vi "造波運動控制.vi"() -> ()   [LabVIEW 2014]
uses:
  <vilib>/Platform/TimedLoop/XDataNode/timing_clust.ctl
  <vilib>/Platform/TimedLoop/XDataNode/nitl_modes.ctl
  <vilib>/Platform/TimedLoop/XDataNode/wakeup.ctl
  <vilib>/Utility/file.llb/Read From Spreadsheet File (DBL).vi
  <vilib>/Utility/file.llb/Write To Spreadsheet File (DBL).vi
  <vilib>/Platform/TimedLoop/XDataNode/XDataNode.xnode
  <vilib>/Platform/TimedLoop/XDataNode/XDNodeRunTimeDep.lvlib
panel:
  out "check trajectory":cluster{"all rows":dbl[], "all rows":dbl[]}[](graph)
  out "imported data 2":cluster{"all rows":dbl[], "all rows":dbl[]}(graph)
  in  "Save file?":bool
  out "new file path (Not A Path if cancelled)":path
  in  "ORG Logic":enum32{"Low Active", "High Active"}(radio)
  in  "Home Mode":u32(ring) items=["MODE1_Abs"=0, "MODE2_Lmt "=1, "MODE3_Ref "=2, "MODE4_Abs_Ref"=3, "MODE5_Abs_NegRef "=4, "MODE6_Lmt_Ref "=5, "MODE7_AbsSearch "=6, "MODE8_LmtSearch"=7, "MODE9_AbsSearch_Ref "=8, "MODE10_AbsSearch_NegRef "=9, "MODE11_LmtSearch_Ref "=10, "MODE12_AbsSearchRefind"=11, "MODE13_LmtSearchRefind"=12, "MODE14_AbsSearchRefind_Ref"=13, "MODE15_AbsSearchRefind_NegRef"=14, "MODE16_LmtSearchRefind_Ref"=15, "CiA402_MODE1"=101, "CiA402_MODE2"=102, "CiA402_MODE3"=103, "CiA402_MODE4"=104, "CiA402_MODE5"=105, "CiA402_MODE6"=106, "CiA402_MODE7"=107, "CiA402_MODE8"=108, "CiA402_MODE9"=109, "CiA402_MODE10"=110, "CiA402_MODE11"=111, "CiA402_MODE12"=112, "CiA402_MODE13"=113, "CiA402_MODE14"=114, "CiA402_MODE15"=115, "CiA402_MODE16"=116, "CiA402_MODE17"=117, "CiA402_MODE18"=118, "CiA402_MODE19"=119, "CiA402_MODE20"=120, "CiA402_MODE21"=121, "CiA402_MODE22"=122, "CiA402_MODE23"=123, "CiA402_MODE24"=124, "CiA402_MODE25"=125, "CiA402_MODE26"=126, "CiA402_MODE27"=127, "CiA402_MODE28"=128, "CiA402_MODE29"=129, "CiA402_MODE30"=130, "CiA402_MODE31"=131, "CiA402_MODE32"=132, "CiA402_MODE33"=133, "CiA402_MODE34"=134, "CiA402_MODE35"=135, "CiA402_MODE36"=136, "CiA402_MODE37"=137]
  in  "Direction":enum32{"Negative", "Positive"}(radio)
  in  "Home":bool
  out "ORG":bool
  out "EZ":bool
  out "HLMT+":bool
  out "HLMT-":bool
  out "Waveform Chart":dbl(graph)
  out "t":dbl[](array[numeric])
  out "xi":dbl[](array[numeric]) format="%#_6f"
  out "Freespace":u16
  out "imported data":cluster{"all rows":dbl[], "all rows":dbl[]}(graph)
  in  "file path (xi)":path=path "C:/Users/NTU WAVES/Desktop/實驗操作/Nwave_Experiment_Xi.txt"
  in  "file path (t)":path=path "C:/Users/NTU WAVES/Desktop/實驗操作/Nwave_Experiment_t.txt"
  in  "import file":bool
  out "Error Code:":u32 format="%x"
  out "Error Msg":string
  out "Error":bool
  in  "Reset Error":bool
  out "Instrument":string="if you want to exit program,please press \"Exit Program\" button"
  out "DeviceNum List":u32[](array[numeric])
  out "Servo_Off":bool
  in  "Servo_On":bool
  in  "Servo On":bool
  out "Axis State:":string
  out "CloseSuccess":bool
  in  "Device Type":u16(ring) items=["PCI-1203-06AE (M0)"]
  out "Ret_GetCommandPosition":u32
  out "Exit Program":bool
  out "DeviceOpened":bool
  out "AxisOpened":bool
  out "AxisHandle_Array":u32[](array[numeric])
  out "DevAxesCount":u32
  out "EmgSucces":bool
  out "DecSuccess":bool
  in  "Stop Mode":enum32{"Dec", "Emg"}(radio)
  in  "Operate Axis":T1(radio)
  in  "Stop":bool
  in  "Move":bool
  out "ResetCounter":bool
  in  "Reset Counter":bool
  out "Axis Position":T2
  out "DeviceHandle":u32
  in  "Stop":bool
  in  "Close Board":bool
  in  "Open Board":bool
  # "Open: Open Board -Servo on\nClose:Servo  off -Close Board"
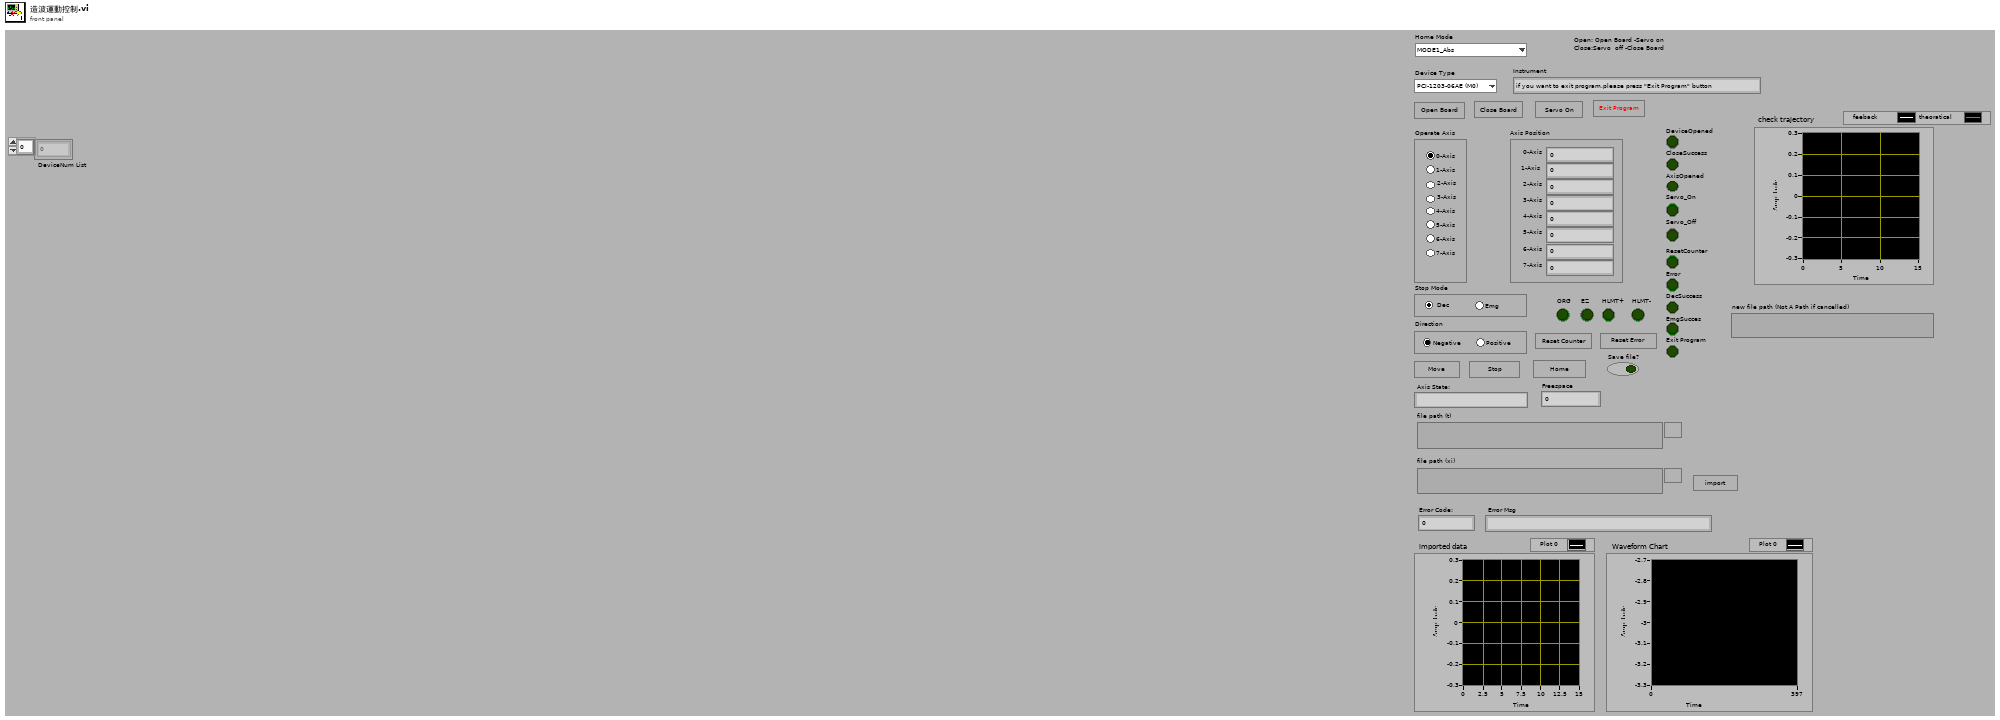
[diagram p1: front panel]
types:
  T1 = enum32{"0-Axis", "1-Axis", "2-Axis", "3-Axis", "4-Axis", "5-Axis", "6-Axis", "7-Axis"}
  T2 = cluster{"0-Axis":dbl, "1-Axis":dbl, "2-Axis":dbl, "3-Axis":dbl, "4-Axis":dbl, "5-Axis":dbl, "6-Axis":dbl, "7-Axis":dbl}
  T3 = cluster{"DeviceNum":u32, "U*8 Array":cluster{"U*8 Array[0]":u8, "U*8 Array[1]":u8, "U*8 Array[2]":u8, "U*8 Array[3]":u8, "U*8 Array[4]":u8, "U*8 Array[5]":u8, "U*8 Array[6]":u8, "U*8 Array[7]":u8, "U*8 Array[8]":u8, "U*8 Array[9]":u8, "U*8 Array[10]":u8, "U*8 Array[11]":u8, "U*8 Array[12]":u8, "U*8 Array[13]":u8, "U*8 Array[14]":u8, "U*8 Array[15]":u8, "U*8 Array[16]":u8, "U*8 Array[17]":u8, "U*8 Array[18]":u8, "U*8 Array[19]":u8, "U*8 Array[20]":u8, "U*8 Array[21]":u8, "U*8 Array[22]":u8, "U*8 Array[23]":u8, "U*8 Array[24]":u8, "U*8 Array[25]":u8, "U*8 Array[26]":u8, "U*8 Array[27]":u8, "U*8 Array[28]":u8, "U*8 Array[29]":u8, "U*8 Array[30]":u8, "U*8 Array[31]":u8, "U*8 Array[32]":u8, "U*8 Array[33]":u8, "U*8 Array[34]":u8, "U*8 Array[35]":u8, "U*8 Array[36]":u8, "U*8 Array[37]":u8, "U*8 Array[38]":u8, "U*8 Array[39]":u8, "U*8 Array[40]":u8, "U*8 Array[41]":u8, "U*8 Array[42]":u8, "U*8 Array[43]":u8, "U*8 Array[44]":u8, "U*8 Array[45]":u8, "U*8 Array[46]":u8, "U*8 Array[47]":u8, "U*8 Array[48]":u8, "U*8 Array[49]":u8}, "NumOfSubDevice":i16}[]
  T4 = cluster{"U*8 Array[0]":u8, "U*8 Array[1]":u8, "U*8 Array[2]":u8, "U*8 Array[3]":u8, "U*8 Array[4]":u8, "U*8 Array[5]":u8, "U*8 Array[6]":u8, "U*8 Array[7]":u8, "U*8 Array[8]":u8, "U*8 Array[9]":u8, "U*8 Array[10]":u8, "U*8 Array[11]":u8, "U*8 Array[12]":u8, "U*8 Array[13]":u8, "U*8 Array[14]":u8, "U*8 Array[15]":u8, "U*8 Array[16]":u8, "U*8 Array[17]":u8, "U*8 Array[18]":u8, "U*8 Array[19]":u8, "U*8 Array[20]":u8, "U*8 Array[21]":u8, "U*8 Array[22]":u8, "U*8 Array[23]":u8, "U*8 Array[24]":u8, "U*8 Array[25]":u8, "U*8 Array[26]":u8, "U*8 Array[27]":u8, "U*8 Array[28]":u8, "U*8 Array[29]":u8, "U*8 Array[30]":u8, "U*8 Array[31]":u8, "U*8 Array[32]":u8, "U*8 Array[33]":u8, "U*8 Array[34]":u8, "U*8 Array[35]":u8, "U*8 Array[36]":u8, "U*8 Array[37]":u8, "U*8 Array[38]":u8, "U*8 Array[39]":u8, "U*8 Array[40]":u8, "U*8 Array[41]":u8, "U*8 Array[42]":u8, "U*8 Array[43]":u8, "U*8 Array[44]":u8, "U*8 Array[45]":u8, "U*8 Array[46]":u8, "U*8 Array[47]":u8, "U*8 Array[48]":u8, "U*8 Array[49]":u8}
  T5 = typedef "XDNodeRunTimeDep.lvlib/timing_clust.ctl" = cluster{"Expected End [f-1]":u64, "Actual End [f-1]":u64, "Finished Late? [f-1]":bool, "Expected End [i-1]":u64, "Actual End [i-1]":u64, "Finished Late? [i-1]":bool, "Expected Start [i]":u64, "Actual Start [i]":u64, "Expected Start [f]":u64, "Actual Start [f]":u64, "Source Name":string, "Structure Name":string, "Period":i64, "Deadline":i64, "Offset":i64, "Start":i64, "Priority":i32, "Timeout":i32, "Mode":T6, "Wakeup Reason":T7, "Error":errorcluster, "Source Type":string, "Secondary Source Type":string, "Global End Time":u64, "Global Start Time":u64, "Frame Duration":u64, "Iteration Duration":u64, "Assigned CPU":i32, "I/O Scan Engine Mode":u32}
  T6 = typedef "XDNodeRunTimeDep.lvlib/nitl_modes.ctl" = enum32{"No Change", "Process missed periods, maintain original phase", "Discard missed periods, maintain original phase", "Process missed periods, ignore original phase", "Discard missed periods, ignore original phase"}
  T7 = typedef "XDNodeRunTimeDep.lvlib/wakeup.ctl" = enum32{"Normal", "Aborted", "Asynchronous wakeup", "Timing source error", "Timed loop error", "Timeout"}
  T8 = cluster{"[0]":dbl, "[1]":dbl, "[2]":dbl, "[3]":dbl, "[4]":dbl, "[5]":dbl, "[6]":dbl, "[7]":dbl}
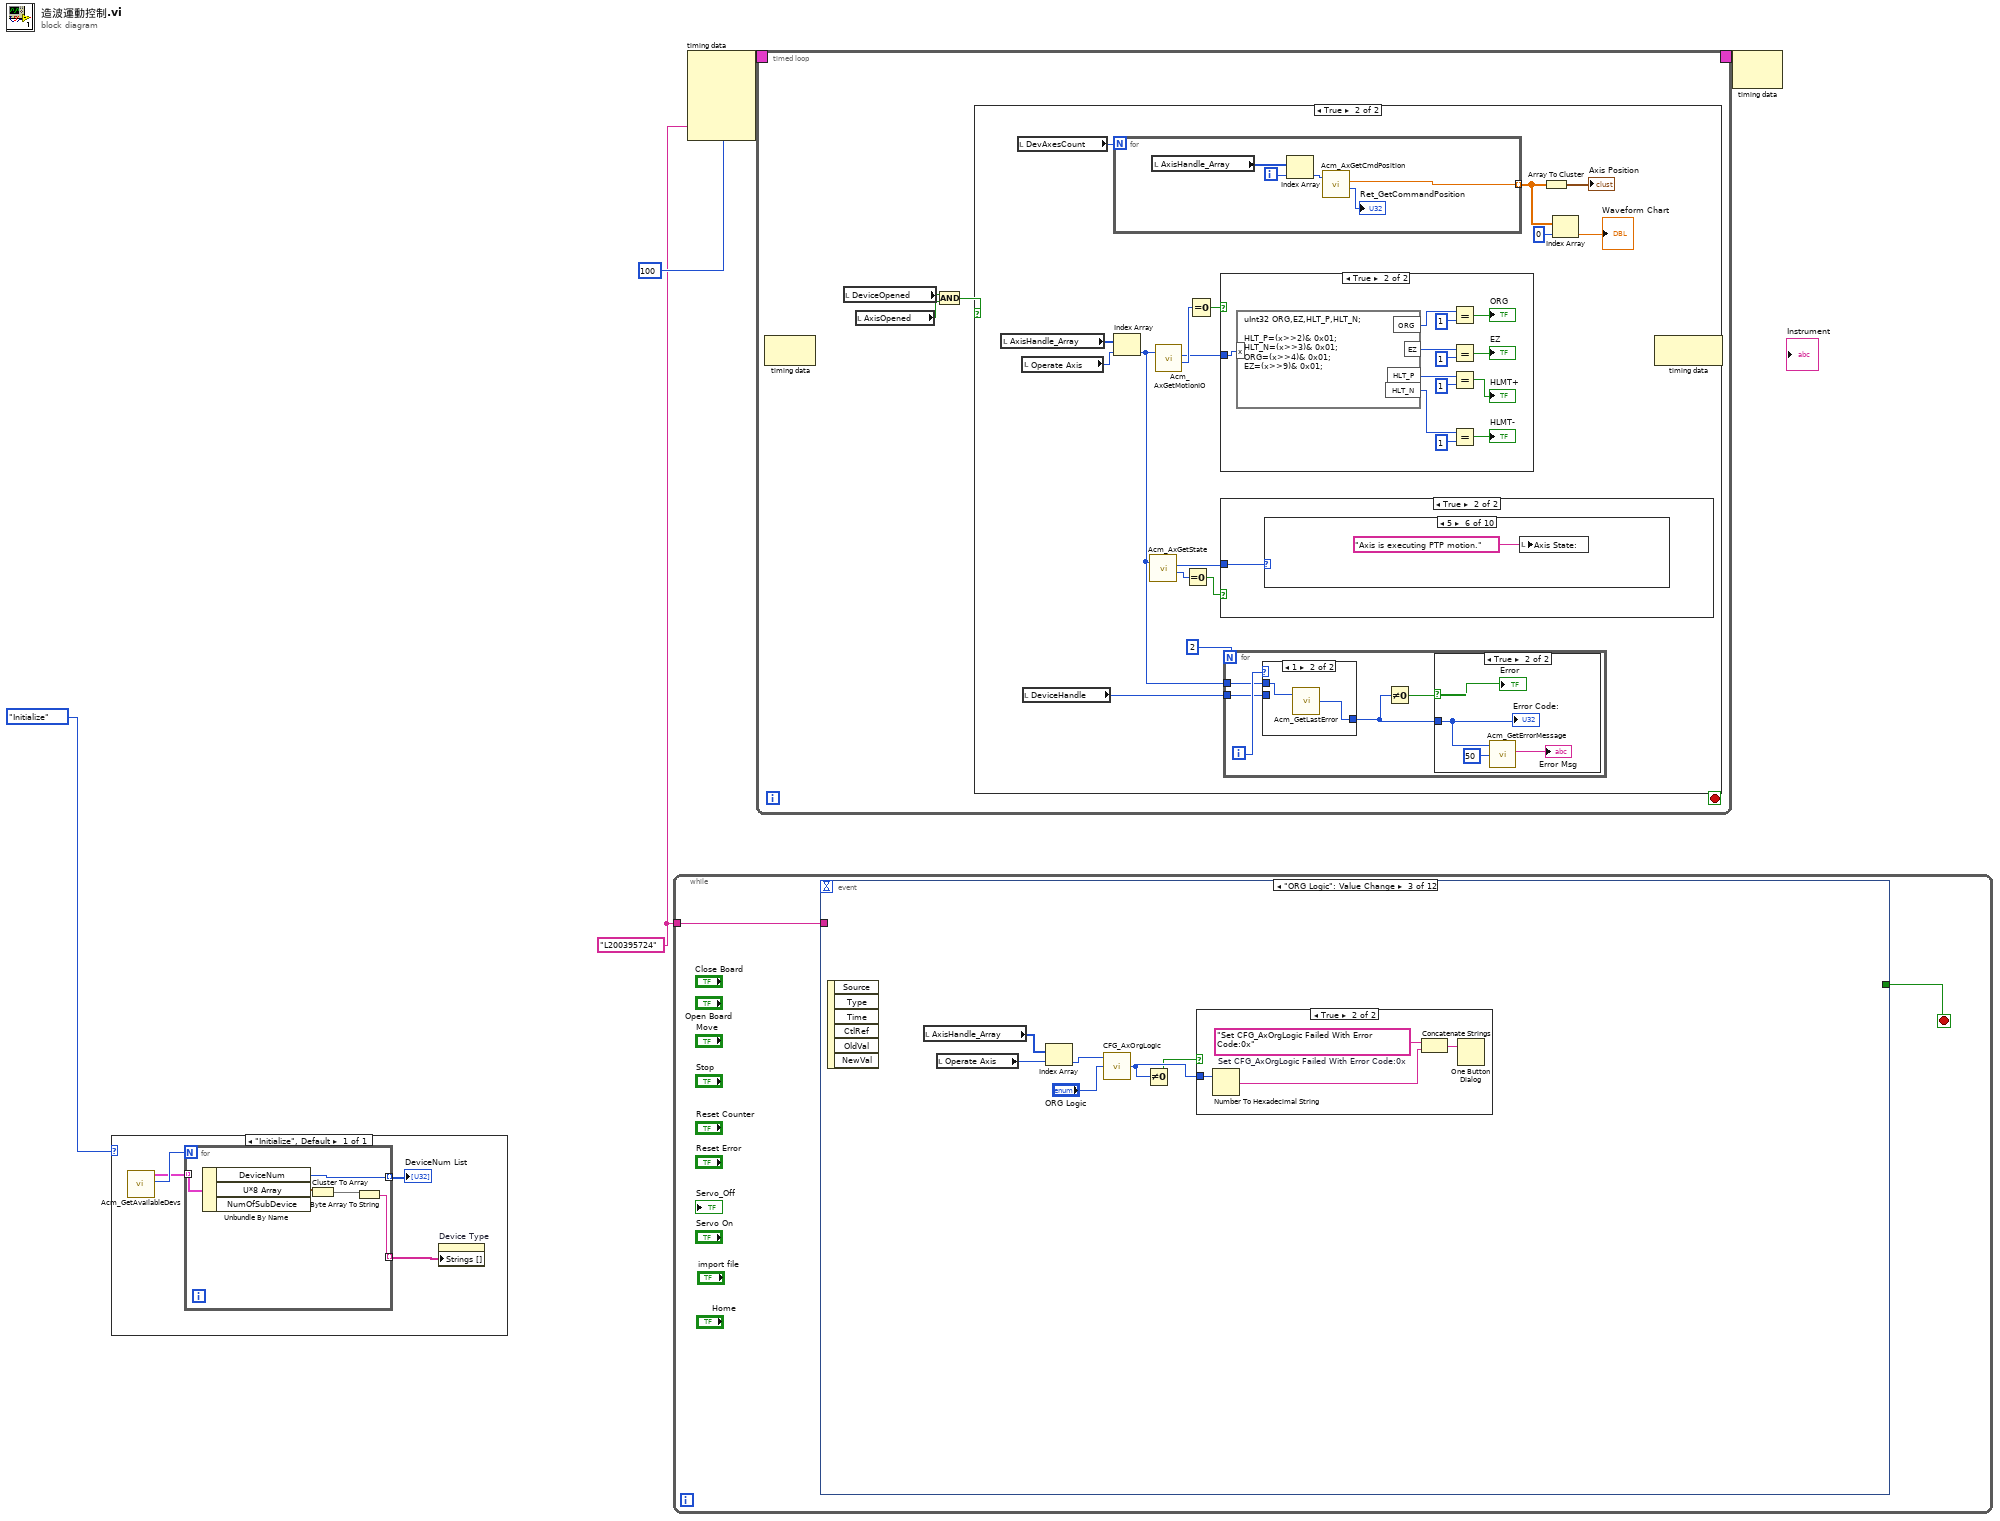
[diagram p0: block diagram]
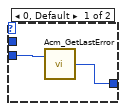
[diagram p5: hidden frame]
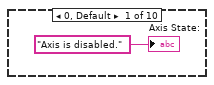
[diagram p7: hidden frame]
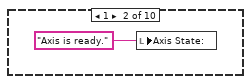
[diagram p8: hidden frame]
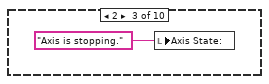
[diagram p9: hidden frame]
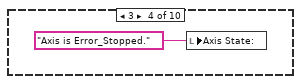
[diagram p10: hidden frame]
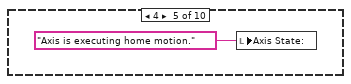
[diagram p11: hidden frame]
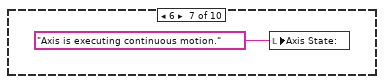
[diagram p12: hidden frame]
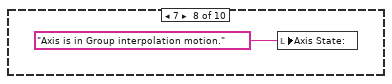
[diagram p13: hidden frame]
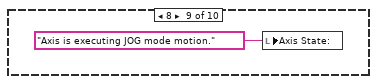
[diagram p14: hidden frame]
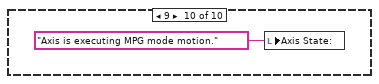
[diagram p15: hidden frame]
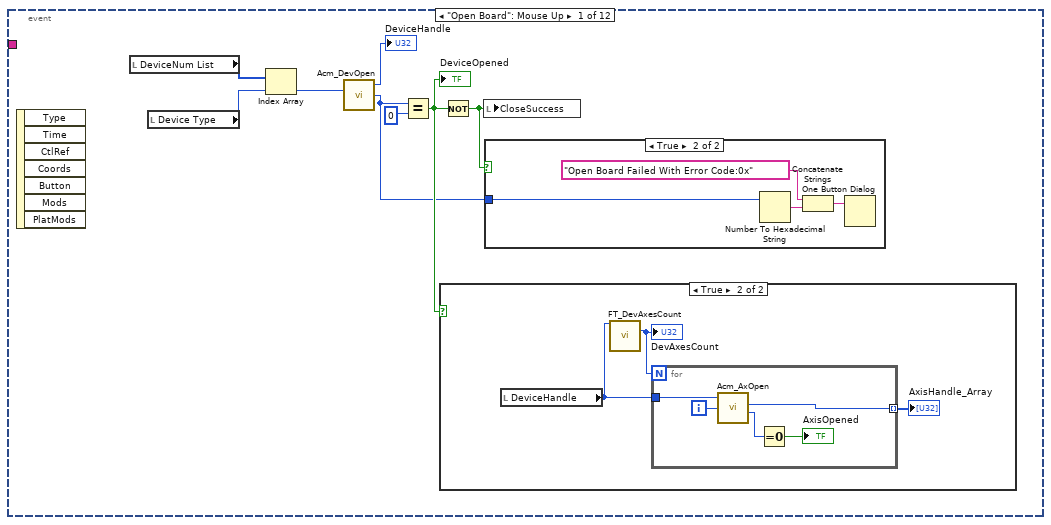
[diagram p16: hidden frame]
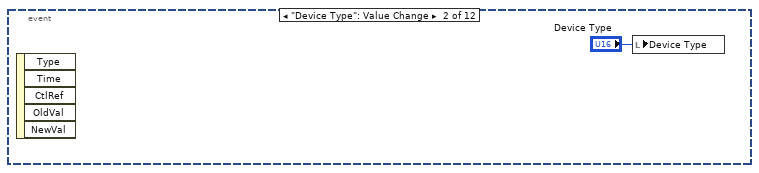
[diagram p19: hidden frame]
diagram:
  w2 = "L200395724" ("结构名称")
  n1 = case shown="\"Initialize\", Default" enum16{"Initialize"}."Initialize" ("Enum") {
    frame "Initialize", Default {
      n2 = call <userlib>:"Acm_GetAvailableDevs.vi"() -> ("DeviceList"=w8:T3, "OutEntries"=w9:u32)  [unwired: 1 in, 4 out]
      n3 = for {
        N: w9 -> [_]
        tunnel: w8 -> [w14] mode=indexing
        tunnel: [w11] -> w7 mode=indexing
        tunnel: [w10] -> w6 mode=indexing
        n4 = Unbundle By Name(w14) -> ("DeviceNum"=w11:u32, "U*8 Array"=w13:T4)  [unwired: 1 out]
        n5 = Cluster To Array(cluster=w13) -> (array=w12:u8[])
        n6 = Byte Array To String(unsigned byte array=w12) -> (string=w10:string)
      }
      "DeviceNum List" <- w7
      n7 = property on="Device Type" class="Ring (strict)"("Strings []"=w6) -> ()  [unwired: 2 in, 2 out]
    }
  }
  n8 = while {
    tunnel: w2 -> [w15]
    stop <- w16 stop-if-true
    n9 = event shown="[2] \"ORG Logic\": Value Change" {
      selector: _ -> [_ _ _ _ _ _ _ _ _ _ _ _]
      dyn-events: _ -> [_ _ _ _ _ _ _ _ _ _ _ _]
      timeout: _ -> [_ _ _ _ _ _ _ _ _ _ _ _]
      tunnel: [_ _ _ _ _ _ _ _ _ _ _ "Stop"] -> w16
      tunnel: w15 -> [_ _ _ _ _ _ _ _ _ _ _ w216]
      event "Open Board": Mouse Up {
        n10 = event-data() -> ()  [unwired: 8 out]
        n11 = local read "DeviceNum List"() -> (w19:u32[])
        n12 = local read "Device Type"() -> (w18:u16)
        n13 = Index Array(array=w19, index=w18) -> (element=w17:u32)
        n14 = call <userlib>:"Acm_DevOpen.vi"("DeviceNumber"=w17) -> ("ReturnValue"=w21:u32, "DeviceHandle"=→"DeviceHandle":u32)  [unwired: 1 in, 1 out]
        n15 = Equal?(x=w21, y=u32 0) -> (x = y?=w22:bool)
        "DeviceOpened" <- w22
        n16 = case shown="True" w22 {
          frame False {
          }
          frame True {
            n17 = local read "DeviceHandle"() -> (w30:u32)
            n18 = call <userlib>:"FT_DevAxesCount.vi"("Handle"=w30) -> ("DevAxesCount"=w31:u32)  [unwired: 1 in, 13 out]
            "DevAxesCount" <- w31
            n19 = for {
              N: w31 -> [_]
              tunnel: w30 -> [w36]
              tunnel: [w32] -> w29 mode=indexing
              i -> [w35]
              n20 = call <userlib>:"Acm_AxOpen.vi"("PhyAxis"=w35, "DeviceHandle"=w36) -> ("ReturnValue"=w34:u32, "AxisHandle"=w32:u32)  [unwired: 1 in, 2 out]
              n21 = Equal To 0?(x=w34) -> (x = 0?=→"AxisOpened":bool)
            }
            "AxisHandle_Array" <- w29
          }
        }
        n22 = Not(x=w22) -> (.not. x?=w20:bool)
        n23 = local write "CloseSuccess"(w20) -> ()
        n24 = case shown="True" w20 {
          tunnel: w21 -> [_ w28]
          frame False {
          }
          frame True {
            n25 = Number To Hexadecimal String(2:w28) -> (0:w26:string)  [unwired: 1 out]
            n26 = Concatenate Strings("Open Board Failed With Error Code:0x", w26) -> (w25:string)
            n27 = One Button Dialog(message=w25) -> ()  [unwired: 2 out]
          }
        }
      }
      event "Device Type": Value Change {
        n28 = event-data() -> ()  [unwired: 6 out]
        n29 = local write "Device Type"("Device Type") -> ()
      }
      event "ORG Logic": Value Change {
        n30 = event-data() -> ()  [unwired: 7 out]
        n31 = local read "AxisHandle_Array"() -> (w42:u32[])
        n32 = local read "Operate Axis"() -> (w41:T1)
        n33 = Index Array(array=w42, index=w41) -> (element=w40:u32)
        n34 = call <userlib>:"CFG_AxOrgLogic.vi"("CFG_AxOrgLogic"="ORG Logic", "Handle"=w40) -> ("ReturnValue"=w39:u32)  [unwired: 1 in, 2 out]
        n35 = Not Equal To 0?(x=w39) -> (x != 0?=w38:bool)
        n36 = case shown="True" w38 {
          tunnel: w39 -> [_ w44]
          frame False {
          }
          frame True {
            w47 = "Set CFG_AxOrgLogic Failed With Error Code:0x"  # Set CFG_AxOrgLogic Failed With Error Code:0x
            n37 = Number To Hexadecimal String(2:w44) -> (0:w46:string)  [unwired: 1 out]
            n38 = Concatenate Strings(w47, w46) -> (w45:string)
            n39 = One Button Dialog(message=w45) -> ()  [unwired: 2 out]
          }
        }
      }
      event "Servo On": Value Change {
        n40 = event-data() -> ()  [unwired: 6 out]
        n41 = local read "AxisHandle_Array"() -> (w57:u32[])
        n42 = local read "Operate Axis"() -> (w56:T1)
        n43 = case shown="True" "Servo_On" {
          tunnel: [u32 1 u32 0] -> w54
          frame False {
          }
          frame True {
          }
        }
        n44 = Index Array(array=w57, index=w56) -> (element=w55:u32)
        n45 = call <userlib>:"Acm_AxSetSvOn.vi"("OnOff"=w54, "AxisHandle"=w55) -> ("ReturnValue"=w48:u32)  [unwired: 1 in, 2 out]
        n46 = local read "Servo On"() -> (w51:bool)
        n47 = Not Equal To 0?(x=w48) -> (x != 0?=w53:bool)
        n48 = Not(x=w53) -> (.not. x?=w52:bool)
        n49 = case shown="True" w53 {
          tunnel: w48 -> [_ w62]
          frame False {
          }
          frame True {
            w65 = "Servo On/Off Failed With Error Code:0x"  # Servo On/Off Failed With Error Code:0x
            n50 = Number To Hexadecimal String(2:w62) -> (0:w64:string)  [unwired: 1 out]
            n51 = Concatenate Strings(w65, w64) -> (w63:string)
            n52 = One Button Dialog(message=w63) -> ()  [unwired: 2 out]
          }
        }
        n53 = And(x=w51, y=w52) -> (x .and. y?=w50:bool)
        n54 = case shown="True" w50 {
          frame False {
            n55 = local write "Servo_On"(FALSE ("Servo_On")) -> ()
            n56 = local write "Servo_Off"(TRUE ("Servo_Off")) -> ()
          }
          frame True {
            n57 = local write "Servo_On"(TRUE ("Servo_On")) -> ()
            n58 = local write "Servo_Off"(FALSE ("Servo_Off")) -> ()
          }
        }
      }
      event "import file": Mouse Up {
        n59 = event-data() -> ()  [unwired: 9 out]
        n60 = local read "AxisHandle_Array"() -> (w85:u32[])
        n61 = local read "Operate Axis"() -> (w69:T1)
        n62 = call-poly <vilib>:"Read From Spreadsheet File.vi"("number of rows (all:-1)"=-1, "file path (dialog if empty)"="file path (t)") -> ("all rows"=w80:dbl[][])  [unwired: 5 in, 4 out]
        n63 = call-poly <vilib>:"Read From Spreadsheet File.vi"("number of rows (all:-1)"=-1, "file path (dialog if empty)"="file path (xi)") -> ("all rows"=w78:dbl[][])  [unwired: 5 in, 4 out]
        n64 = Index Array(array=w85, index=w69) -> (element=w76:u32)
        n65 = Index Array(array=w80, index (col)=0 ("disabled index (col)")) -> (element=w71:dbl[])  [unwired: 1 in]
        "t" <- w71
        n66 = Index Array(array=w78, index (col)=0 ("disabled index (col)")) -> (element=w70:dbl[])  [unwired: 1 in]
        "xi" <- w70
        n67 = call <userlib>:"Acm_AxCheckPTBuffer.vi"("AxisHandle"=w76) -> ("Freespace"=→"Freespace":u16, "ReturnValue"=w74:u32)  [unwired: 1 in, 2 out]
        n68 = Equal To 0?(x=w74) -> (x = 0?=w73:bool)
        n69 = Bundle("all rows"=w71, "all rows"=w70) -> (→"imported data":cluster{"all rows":dbl[], "all rows":dbl[]})  [unwired: 1 in]
        n70 = Not(x=w73) -> (.not. x?=w72:bool)
        n71 = case shown="True" w72 {
          tunnel: w74 -> [_ w86]
          frame False {
          }
          frame True {
            n72 = Number To Hexadecimal String(2:w86) -> (0:w88:string)  [unwired: 1 out]
            n73 = Concatenate Strings("PTBuffer Absolutely Failed With Error Code:0x", w88) -> (w87:string)
            n74 = One Button Dialog(message=w87) -> ()  [unwired: 2 out]
          }
        }
      }
      event "Move": Mouse Up {
        n75 = event-data() -> ()  [unwired: 9 out]
        n76 = local read "AxisHandle_Array"() -> (w112:u32[])
        n77 = local read "t"() -> (w100:dbl[])
        n78 = local read "xi"() -> (w111:dbl[])
        n79 = Index Array(array=w112, index="Operate Axis") -> (element=w104:u32)
        n80 = Multiply(x=w100, y=1000) -> (x*y=w95:dbl[])
        n81 = Multiply(x=100000, y=w111) -> (x*y=w96:dbl[])
        n82 = Bundle(w95, w96) -> (→"imported data 2":cluster{dbl[], dbl[]})  [unwired: 1 in]
        n83 = Tick Count (ms)() -> (millisecond timer value=w105:u32)
        n84 = for {
          tunnel: w104 -> [w137]
          tunnel: w96 -> [w136] mode=indexing
          tunnel: w95 -> [w135] mode=indexing
          n85 = call <userlib>:"Acm_AxAddPTData.vi"("Time"=w135, "Position"=w136, "AxisHandle"=w137) -> ("AxisHandle"=w138:u32)  [unwired: 1 in, 2 out]
          n86 = call <userlib>:"Acm_AxStartPT.vi"("AxisHandle"=w138) -> ()  [unwired: 2 in, 3 out]
        }
        n87 = Array Size(array=w100) -> (size(s)=w107:i32)
        n88 = Decrement(x=w107) -> (x-1=w106:i32)
        n89 = Index Array(array=w95, index=w106) -> (element=w102:dbl)
        n90 = while {
          tunnel: w102 -> [w131]
          shift-right: [w129] -> w93
          shift-left: dbl[] [] -> [w130]
          tunnel: w105 -> [w127]
          tunnel: w104 -> [w126]
          shift-right: [w125] -> w94
          shift-left: dbl[] [] -> [w124]
          i -> [w123]
          stop <- w133 stop-if-true
          w122 = u32 10 ("millisecond multiple")
          n91 = call <userlib>:"Acm_AxGetActualPosition.vi"("AxisHandle"=w126) -> ("Position"=w128:dbl)  [unwired: 1 in, 3 out]
          n92 = Multiply(x=w123, y=w122) -> (x*y=w120:u32)
          n93 = Tick Count (ms)() -> (millisecond timer value=w134:u32)
          n94 = Divide(x=w128, y=100000.0) -> (x/y=w118:dbl)
          n95 = Divide(x=w120, y=u32 1000) -> (x/y=w121:dbl)
          n96 = Subtract(x=w134, y=w127) -> (x-y=w132:u32)
          n97 = Wait Until Next ms Multiple(millisecond multiple=w122) -> ()  [unwired: 1 out]
          n98 = Insert Into Array(array=w130, new element=w118) -> (w129:dbl[])  [unwired: 1 in]
          n99 = Greater Or Equal?(x=w132, y=w131) -> (x >= y?=w133:bool)
          n100 = Insert Into Array(array=w124, new element=w121) -> (w125:dbl[])  [unwired: 1 in]
        }
        n101 = local read "imported data"() -> (w91:cluster{"all rows":dbl[], "all rows":dbl[]})
        n102 = Build Array(w94, w93) -> (w98:dbl[][])
        n103 = Bundle(w94, w93) -> (w92:cluster{dbl[], dbl[]})  [unwired: 1 in]
        n104 = case shown="True" "Save file?" {
          tunnel: w98 -> [_ w115]
          frame False {
          }
          frame True {
            n105 = call-poly <vilib>:"Write To Spreadsheet File.vi"("delimiter (\\t)"="," ("delimiter (\\t)"), "transpose? (no:F)"=TRUE, "2D data"=w115) -> ("new file path (Not A Path if cancelled)"=→"new file path (Not A Path if cancelled)":path)  [unwired: 5 in]
          }
        }
        n106 = Build Array(w92, w91) -> (→"check trajectory":cluster{"all rows":dbl[], "all rows":dbl[]}[])
      }
      event "Stop": Mouse Up {
        n107 = event-data() -> ()  [unwired: 8 out]
        n108 = local read "AxisHandle_Array"() -> (w142:u32[])
        n109 = local read "Operate Axis"() -> (w140:T1)
        n110 = Index Array(array=w142, index=w140) -> (element=w141:u32)
        n111 = case shown="\"Emg\"" "Stop Mode" {
          tunnel: w141 -> [w145 w154]
          frame "Dec", Default {
            n112 = call <userlib>:"Acm_AxStopDec.vi"("AxisHandle"=w145) -> ("ReturnValue"=w146:u32)  [unwired: 1 in, 2 out]
            n113 = Equal To 0?(x=w146) -> (x = 0?=w144:bool)
            "DecSuccess" <- w144
            n114 = Not(x=w144) -> (.not. x?=w143:bool)
            n115 = case shown="True" w143 {
              tunnel: w145 -> [_ w150]
              frame False {
              }
              frame True {
                n116 = Number To Hexadecimal String(2:w150) -> (0:w148:string)  [unwired: 1 out]
                n117 = Concatenate Strings("Stop Failed With Error Code:0x", w148) -> (w147:string)
                n118 = One Button Dialog(message=w147) -> ()  [unwired: 2 out]
              }
            }
          }
          frame "Emg" {
            n119 = call <userlib>:"Acm_AxStopEmg.vi"("AxisHandle"=w154) -> ("ReturnValue"=w151:u32)  [unwired: 1 in, 2 out]
            n120 = Equal To 0?(x=w151) -> (x = 0?=w153:bool)
            "EmgSucces" <- w153
            n121 = Not(x=w153) -> (.not. x?=w152:bool)
            n122 = case shown="True" w152 {
              tunnel: w151 -> [_ w158]
              frame False {
              }
              frame True {
                n123 = Number To Hexadecimal String(2:w158) -> (0:w156:string)  [unwired: 1 out]
                n124 = Concatenate Strings("Stop failed with Error Code:0x", w156) -> (w155:string)
                n125 = One Button Dialog(message=w155) -> ()  [unwired: 2 out]
              }
            }
          }
        }
      }
      event "Home": Mouse Up {
        n126 = event-data() -> ()  [unwired: 9 out]
        n127 = local read "AxisHandle_Array"() -> (w161:u32[])
        n128 = local read "Operate Axis"() -> (w160:T1)
        n129 = Index Array(array=w161, index=w160) -> (element=w159:u32)
        n130 = case shown="\"Positive\"" "Direction" {
          tunnel: w159 -> [w163 w173]
          frame "Negative", Default {
            n131 = call <userlib>:"Acm_AxHome.vi"("DirMode"=u32 1, "HomeMode"="Home Mode", "AxisHandle"=w163) -> ("ReturnValue"=w166:u32)  [unwired: 1 in, 2 out]
            n132 = Equal To 0?(x=w166) -> (x = 0?=w167:bool)
            n133 = Not(x=w167) -> (.not. x?=w168:bool)
            n134 = case shown="True" w168 {
              tunnel: w166 -> [_ w169]
              frame False {
              }
              frame True {
                n135 = Number To Hexadecimal String(2:w169) -> (0:w171:string)  [unwired: 1 out]
                n136 = Concatenate Strings("Go Home failed with Error Code:0x", w171) -> (w170:string)
                n137 = One Button Dialog(message=w170) -> ()  [unwired: 2 out]
              }
            }
          }
          frame "Positive" {
            n138 = local read "Home Mode"() -> (w175:u32)
            n139 = call <userlib>:"Acm_AxHome.vi"("DirMode"=u32 0, "HomeMode"=w175, "AxisHandle"=w173) -> ("ReturnValue"=w177:u32)  [unwired: 1 in, 2 out]
            n140 = Not Equal To 0?(x=w177) -> (x != 0?=w176:bool)
            n141 = case shown="True" w176 {
              tunnel: w177 -> [_ w178]
              frame False {
              }
              frame True {
                n142 = Number To Hexadecimal String(2:w178) -> (0:w180:string)  [unwired: 1 out]
                n143 = Concatenate Strings("Go Home Failed With Error Code:0x", w180) -> (w179:string)
                n144 = One Button Dialog(message=w179) -> ()  [unwired: 2 out]
              }
            }
          }
        }
      }
      event "Reset Counter": Mouse Up {
        n145 = event-data() -> ()  [unwired: 8 out]
        n146 = local read "AxisOpened"() -> (w182:bool)
        n147 = case shown="True" w182 {
          frame False {
          }
          frame True {
            n148 = local read "DevAxesCount"() -> (w183:u32)
            n149 = for {
              N: w183 -> [_]
              i -> [w188]
              n150 = local read "AxisHandle_Array"() -> (w189:u32[])
              n151 = Index Array(array=w189, index=w188) -> (element=w187:u32)
              n152 = call <userlib>:"Acm_AxSetCmdPosition.vi"("Position"=0.0, "AxisHandle"=w187) -> ("ReturnValue"=w185:u32)  [unwired: 1 in, 2 out]
              n153 = Equal To 0?(x=w185) -> (x = 0?=→"ResetCounter":bool)
            }
          }
        }
      }
      event "Reset Error": Mouse Up {
        n154 = event-data() -> ()  [unwired: 9 out]
        n155 = local read "AxisOpened"() -> (w190:bool)
        n156 = case shown="True" w190 {
          frame False {
          }
          frame True {
            n157 = local read "AxisHandle_Array"() -> (w193:u32[])
            n158 = local read "Operate Axis"() -> (w191:T1)
            n159 = Index Array(array=w193, index=w191) -> (element=w192:u32)
            n160 = call <userlib>:"Acm_AxResetError.vi"("AxisHandle"=w192) -> ()  [unwired: 1 in, 3 out]
          }
        }
      }
      event "Close Board": Mouse Up {
        n161 = event-data() -> ()  [unwired: 8 out]
        n162 = stacked-sequence {
          frame #0 {
            n163 = local read "DevAxesCount"() -> (w194:u32)
            n164 = for {
              N: w194 -> [_]
              i -> [w199]
              n165 = local read "AxisHandle_Array"() -> (w200:u32[])
              n166 = Index Array(array=w200, index=w199) -> (element=w198:u32)
              n167 = call <userlib>:"Acm_AxClose.vi"("AxisHandle"=w198) -> ("ReturnValue"=w197:u32)  [unwired: 1 in, 1 out]
              n168 = Equal To 0?(x=w197) -> (x = 0?=w196:bool)
              n169 = Not(x=w196) -> (.not. x?=w195:bool)
              n170 = local write "AxisOpened"(w195) -> ()
            }
          }
          frame #1 {
            n171 = local read "DeviceHandle"() -> (w204:u32)
            n172 = call <userlib>:"Acm_DevClose.vi"("DeviceHandle"=w204) -> ("ReturnValue"=w203:u32)  [unwired: 1 in, 3 out]
            n173 = Equal To 0?(x=w203) -> (x = 0?=w202:bool)
            "CloseSuccess" <- w202
            n174 = Not(x=w202) -> (.not. x?=w201:bool)
            n175 = case shown="True" w202 {
              tunnel: w202 -> [_ w210]
              frame False {
              }
              frame True {
                n176 = Not(x=w210) -> (.not. x?=w209:bool)
                n177 = local write "DevAxesCount"(u32 0 ("DevAxesCount")) -> ()
                n178 = local write "DeviceHandle"(u32 0 ("DeviceHandle")) -> ()
                n179 = local write "DeviceOpened"(w209) -> ()
                n180 = local write "EmgSucces"(w209) -> ()
                n181 = local write "DecSuccess"(w209) -> ()
                n182 = local write "ResetCounter"(w209) -> ()
                n183 = local read "DevAxesCount"() -> (w213:u32)
                n184 = Initialize Array(u32 0 ("元素"), w213) -> (w212:u32[])
                n185 = local write "AxisHandle_Array"(w212) -> ()
              }
            }
            n186 = case shown="True" w201 {
              tunnel: w203 -> [_ w208]
              frame False {
              }
              frame True {
                n187 = Number To Hexadecimal String(2:w208) -> (0:w206:string)  [unwired: 1 out]
                n188 = Concatenate Strings("Close Board Failed With Error Code:0x", w206) -> (w205:string)
                n189 = One Button Dialog(message=w205) -> ()  [unwired: 2 out]
              }
            }
          }
        }
      }
      event "Stop": Value Change {
        n190 = event-data() -> ()  [unwired: 6 out]
        n191 = call <vilib>:"Stop Timed Structure.vi"("name"=w216) -> ()  [unwired: 2 in, 9 out]
        "Exit Program" <- "Stop"
      }
    }
  }
  n192 = node-c288(i64 100 ("周期"), w2) -> (w5:T5)  [unwired: 3 out]
  n193 = timed-loop {
    timing: w5 -> [_]
    timing-out: [_] -> w4
    stop <- _ stop-if-true
    n194 = node-c288() -> ()  [unwired: 2 out]
    n195 = local read "DeviceOpened"() -> (w219:bool)
    n196 = local read "AxisOpened"() -> (w220:bool)
    n197 = And(x=w219, y=w220) -> (x .and. y?=w218:bool)
    n198 = case shown="True" w218 {
      frame False {
      }
      frame True {
        n199 = local read "AxisHandle_Array"() -> (w234:u32[])
        n200 = local read "DevAxesCount"() -> (w235:u32)
        n201 = local read "Operate Axis"() -> (w233:T1)
        n202 = local read "DeviceHandle"() -> (w228:u32)
        n203 = for {
          N: w235 -> [_]
          tunnel: [w275] -> w227 mode=indexing
          i -> [w277]
          n204 = local read "AxisHandle_Array"() -> (w278:u32[])
          n205 = Index Array(array=w278, index=w277) -> (element=w276:u32)
          n206 = call <userlib>:"Acm_AxGetCmdPosition.vi"("AxisHandle"=w276) -> ("ReturnValue"=→"Ret_GetCommandPosition":u32, "Position"=w275:dbl)  [unwired: 1 in, 2 out]
        }
        n207 = Index Array(array=w234, index=w233) -> (element=w224:u32)
        n208 = call <userlib>:"Acm_AxGetState.vi"("AxisHandle"=w224) -> ("ReturnValue"=w232:u32, "Status"=w230:u16)  [unwired: 1 in, 2 out]
        n209 = call <userlib>:"Acm_AxGetMotionIO.vi"("AxisHandle"=w224) -> ("ReturnValue"=w222:u32, "Status"=w221:u32)  [unwired: 1 in, 2 out]
        n210 = Equal To 0?(x=w232) -> (x = 0?=w231:bool)
        n211 = Equal To 0?(x=w222) -> (x = 0?=w223:bool)
        n212 = case shown="True" w223 {
          tunnel: w221 -> [_ w237]
          frame False {
          }
          frame True {
            n213 = formula code="uInt32 ORG,EZ,HLT_P,HLT_N;\n\nHLT_P=(x>>2)& 0x01;\nHLT_N=(x>>3)& 0x01;\nORG=(x>>4)& 0x01;\nEZ=(x>>9)& 0x01;"("x"=w237) -> ("ORG"=w248:u32, "EZ"=w246:u32, "HLT_P"=w244:u32, "HLT_N"=w239:u32)
            n214 = Equal?(x=w248, y=u32 1) -> (x = y?=→"ORG":bool)
            n215 = Equal?(x=w246, y=u32 1) -> (x = y?=→"EZ":bool)
            n216 = Equal?(x=w244, y=u32 1) -> (x = y?=→"HLMT+":bool)
            n217 = Equal?(x=w239, y=u32 1) -> (x = y?=→"HLMT-":bool)
          }
        }
        n218 = case shown="True" w231 {
          tunnel: w230 -> [_ w263]
          frame False {
          }
          frame True {
            n219 = case shown="5" w263 {
              frame 0, Default {
                "Axis State:" <- "Axis is disabled." ("Axis State:")
              }
              frame 1 {
                n220 = local write "Axis State:"("Axis is ready." ("Axis State:")) -> ()
              }
              frame 2 {
                n221 = local write "Axis State:"("Axis is stopping." ("Axis State:")) -> ()
              }
              frame 3 {
                n222 = local write "Axis State:"("Axis is Error_Stopped." ("Axis State:")) -> ()
              }
              frame 4 {
                n223 = local write "Axis State:"("Axis is executing home motion." ("Axis State:")) -> ()
              }
              frame 5 {
                n224 = local write "Axis State:"("Axis is executing PTP motion." ("Axis State:")) -> ()
              }
              frame 6 {
                n225 = local write "Axis State:"("Axis is executing continuous motion." ("Axis State:")) -> ()
              }
              frame 7 {
                n226 = local write "Axis State:"("Axis is in Group interpolation motion." ("Axis State:")) -> ()
              }
              frame 8 {
                n227 = local write "Axis State:"("Axis is executing JOG mode motion." ("Axis State:")) -> ()
              }
              frame 9 {
                n228 = local write "Axis State:"("Axis is executing MPG mode motion." ("Axis State:")) -> ()
              }
            }
          }
        }
        n229 = for {
          N: 2 -> [_]
          tunnel: w228 -> [w253]
          tunnel: w224 -> [w252]
          i -> [w254]
          n230 = case shown="1" w254 {
            tunnel: [w260 w262] -> w251
            tunnel: w253 -> [w259 _]
            tunnel: w252 -> [_ w261]
            frame 0, Default {
              n231 = call <userlib>:"Acm_GetLastError.vi"("ObjectHandle"=w259) -> ("ReturnValue"=w260:u32)  [unwired: 1 in, 2 out]
            }
            frame 1 {
              n232 = call <userlib>:"Acm_GetLastError.vi"("ObjectHandle"=w261) -> ("ReturnValue"=w262:u32)  [unwired: 1 in, 2 out]
            }
          }
          n233 = Not Equal To 0?(x=w251) -> (x != 0?=w250:bool)
          n234 = case shown="True" w250 {
            selector: w250 -> [_ w257]
            tunnel: w251 -> [_ w256]
            frame False {
            }
            frame True {
              n235 = call <userlib>:"Acm_GetErrorMessage.vi"("nMaxError"=50, "ErrorCode"=w256) -> ("ErrorMsg"=→"Error Msg":string)  [unwired: 4 out]
              "Error" <- w257
              "Error Code:" <- w256
            }
          }
        }
        n236 = Array To Cluster(array=w227) -> (cluster=→"Axis Position":T8)
        n237 = Index Array(array=w227, index=0) -> (element=→"Waveform Chart":dbl)
      }
    }
    n238 = node-c288() -> ()  [unwired: 2 out]
  }
  n239 = node-c288(w4) -> ()  [unwired: 1 out]
